vi "write-log.vi"(10 "Write Text":string, 11 "Internal Cluster":T1) -> ()   [LabVIEW 2015]
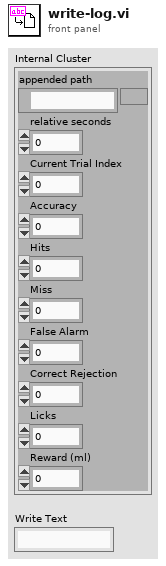
[diagram p1: front panel]
types:
  T1 = cluster{"appended path":path, "relative seconds":dbl, "Current Trial Index":i32, "Accuracy":i32, "Hits":i32, "Miss":i32, "False Alarm":i32, "Correct Rejection":i32, "Licks":i32, "Reward (ml)":i32}
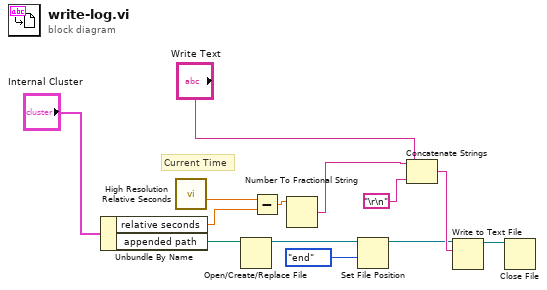
[diagram p0: block diagram]
diagram:
  # "Current Time"
  n1 = Unbundle By Name("Internal Cluster") -> ("relative seconds"=w13:dbl, "appended path"=w8:path)
  n2 = call <vilib>:"High Resolution Relative Seconds.vi"() -> ("relative seconds"=w2:dbl)
  n3 = Open/Create/Replace File(file path (use dialog)=w8) -> (refnum out=w9:refnum<file>)  [unwired: 5 in, 2 out]
  n4 = Subtract(x=w2, y=w13) -> (x-y=w5:dbl)
  n5 = Number To Fractional String(number=w5) -> (F-format string=w6:string)  [unwired: 3 in]
  n6 = Set File Position(refnum=w9, from (0:start)=enum16{"start", "end", "current"}."end") -> (refnum out=w11:refnum<file>)  [unwired: 2 in, 1 out]
  n7 = Concatenate Strings(w6, "Write Text", "\r\n") -> (w12:string)
  n8 = Write to Text File(file (use dialog)=w11, text=w12) -> (refnum out=w7:refnum<file>)  [unwired: 2 in, 2 out]
  n9 = Close File(refnum=w7) -> ()  [unwired: 1 in, 2 out]
